vi "EnqueueSub.vi"(5 "is valid (T)":bool, 6 "is last element (F)":bool, 7 "nonFull":refnum<k4>, 8 "element in":T1, 9 "size":i32, 10 "lastID":u32, 11 "SubChannel in":refnum<class "SubChannelCPU.lvclass">) -> (0 "element out":T1, 1 "count":i32, 2 "wait":bool, 3 "SubChannel out":refnum<class "SubChannelCPU.lvclass">, 4 "id":u32)   [LabVIEW 2019, in "MessengerM.lvlib" / "SubChannelCPU.lvclass"]
uses:
  SubChannelCPU.lvclass
  <resource>/ChannelSupport/_ChannelSupport/PipeLogic2/PipeLogic2.lvclass
  Element.ctl
  MessengerM.lvlib
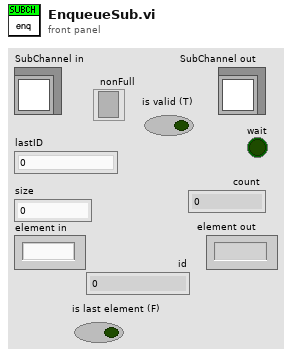
[diagram p1: front panel]
types:
  T1 = typedef "MessengerM.lvlib/Element.ctl" = string
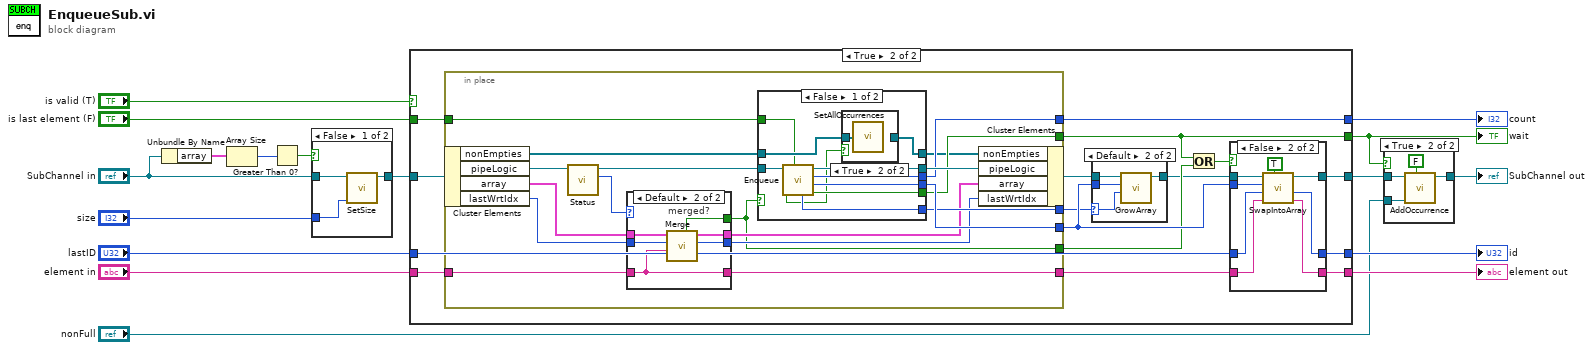
[diagram p0: block diagram]
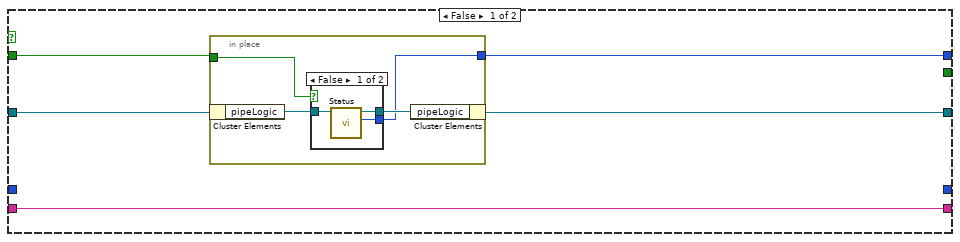
[diagram p2: hidden frame]
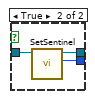
[diagram p3: hidden frame]
diagram:
  n1 = Unbundle By Name("SubChannel in") -> ("array"=w15:cluster{"elt":T1}[])
  n2 = Array Size(array=w15) -> (size(s)=w14:i32)
  n3 = Greater Than 0?(x=w14) -> (x > 0?=w16:bool)
  n4 = case shown="False" w16 {
    tunnel: "SubChannel in" -> [w20 w21]
    tunnel: [w19 w21] -> w17
    tunnel: "size" -> [w18 _]
    frame False {
      n5 = call "SetSize.vi"("size"=w18, "SubChannel in"=w20) -> ("SubChannel out"=w19:refnum<class "SubChannelCPU.lvclass">)  [unwired: 9 in]
    }
    frame True {
    }
  }
  n6 = case shown="True" "is valid (T)" {
    tunnel: w17 -> [w25 w51]
    tunnel: "element in" -> [w26 w44]
    tunnel: [w26 w43] -> w11
    tunnel: [w22 w42] -> w10
    tunnel: "lastID" -> [_ w41]
    tunnel: [_ w40] -> w8
    tunnel: [w24 w39] -> w7
    tunnel: [_ w38] -> w3
    tunnel: "is last element (F)" -> [w23 w37]
    frame False {
      n7 = in-place {
        in-place-border: w23 -> [w30]
        in-place-border: [w27] -> w22
        n8 = in-place-cluster #1(w25) -> ("pipeLogic"=w29:refnum<class "PipeLogic2.lvclass">)
        n9 = case shown="False" w30 {
          tunnel: w29 -> [w33 w36]
          tunnel: [w32 w35] -> w28
          tunnel: [w31 w34] -> w27
          frame False {
            n10 = call <resource>:"Status.vi"("pipeLogic in"=w33) -> ("count"=w31:i32, "pipeLogic out"=w32:refnum<class "PipeLogic2.lvclass">)  [unwired: 4 in, 5 out]
          }
          frame True {
            n11 = call <resource>:"SetSentinel.vi"("pipeLogic in"=w36) -> ("count"=w34:i32, "pipeLogic out"=w35:refnum<class "PipeLogic2.lvclass">)  [unwired: 8 in, 1 out]
          }
        }
        n12 = in-place-cluster #1("pipeLogic"=w28) -> (w24:refnum<class "SubChannelCPU.lvclass">)
      }
    }
    frame True {
      n13 = in-place {
        in-place-border: [w69] -> w42
        in-place-border: [w68] -> w52
        in-place-border: [w66] -> w47
        in-place-border: [w67] -> w38
        in-place-border: w44 -> [w60]
        in-place-border: [w59] -> w48
        in-place-border: [w56] -> w50
        in-place-border: w37 -> [w53]
        n14 = in-place-cluster #2(w51) -> ("nonEmpties"=w55:refnum<k4>[], "pipeLogic"=w65:refnum<class "PipeLogic2.lvclass">, "array"=w61:cluster{"elt":T1}[], "lastWrtIdx"=w58:i32)
        n15 = call <resource>:"Status.vi"("pipeLogic in"=w65) -> ("count"=w63:i32, "pipeLogic out"=w64:refnum<class "PipeLogic2.lvclass">)  [unwired: 4 in, 5 out]
        n16 = case shown="Default" w63 {
          tunnel: [w73 w76] -> w62
          tunnel: w61 -> [w73 w79]
          tunnel: w60 -> [w72 w78]
          tunnel: [_ w75] -> w56
          tunnel: [w72 w78] -> w59
          tunnel: w58 -> [w71 w77]
          tunnel: [w71 w74] -> w57
          frame 0 {
          }
          frame Default {
            # "merged?"
            n17 = call "Merge.vi"("element in"=w78, "lastWrtIdx in"=w77, "array in"=w79) -> ("lastWrtIdx out"=w74:i32, "array out"=w76:cluster{"elt":T1}[], "merged?"=w75:bool)  [unwired: 6 in]
          }
        }
        n18 = case shown="False" w56 {
          tunnel: [w89 w93] -> w70
          tunnel: [w88 _] -> w69
          tunnel: [w87 _] -> w68
          tunnel: [w86 _] -> w67
          tunnel: [w85 _] -> w66
          tunnel: w64 -> [w84 w93]
          tunnel: w55 -> [w82 w92]
          tunnel: [w81 w92] -> w54
          tunnel: w53 -> [w80 _]
          frame False {
            n19 = call <resource>:"Enqueue.vi"("last element in"=w80, "pipeLogic in"=w84) -> ("wait"=w86:bool, "index"=w87:i32, "count"=w88:i32, "pipeLogic out"=w89:refnum<class "PipeLogic2.lvclass">, "grow"=w85:i32, "set nonempty"=w83:bool)  [unwired: 2 in, 2 out]
            n20 = case shown="True" w83 {
              tunnel: w82 -> [w90 w91]
              tunnel: [w90 _] -> w81
              frame False {
              }
              frame True {
                n21 = call "SetAllOccurrences.vi"("occurrences"=w91) -> ()
              }
            }
          }
          frame True {
          }
        }
        n22 = in-place-cluster #2("nonEmpties"=w54, "pipeLogic"=w70, "array"=w62, "lastWrtIdx"=w57) -> (w45:refnum<class "SubChannelCPU.lvclass">)
      }
      n23 = case shown="Default" w47 {
        selector: w47 -> [_ w96]
        tunnel: w45 -> [w94 w98]
        tunnel: [w94 w97] -> w46
        tunnel: w52 -> [_ w95]
        frame 0 {
        }
        frame Default {
          n24 = call "GrowArray.vi"("grow"=w96, "index"=w95, "SubChannel in"=w98) -> ("SubChannel out"=w97:refnum<class "SubChannelCPU.lvclass">)  [unwired: 8 in]
        }
      }
      n25 = Or(x=w38, y=w50) -> (x .or. y?=w49:bool)
      n26 = case shown="False" w49 {
        tunnel: [w100 w108] -> w39
        tunnel: [w101 w106] -> w43
        tunnel: w48 -> [w101 w107]
        tunnel: w46 -> [w100 w109]
        tunnel: [w99 w104] -> w40
        tunnel: w52 -> [_ w103]
        tunnel: w41 -> [w99 w102]
        frame True {
          # "wait"
        }
        frame False {
          n27 = call "SwapIntoArray.vi"("enq"=TRUE, "element in"=w107, "last id"=w102, "index"=w103, "SubChannel in"=w109) -> ("element out"=w106:T1, "id"=w104:u32, "SubChannel out"=w108:refnum<class "SubChannelCPU.lvclass">)  [unwired: 4 in]
        }
      }
    }
  }
  "element out" <- w11
  "wait" <- w3
  "count" <- w10
  "id" <- w8
  n28 = case shown="True" w3 {
    tunnel: w7 -> [w110 w114]
    tunnel: [w110 w113] -> w6
    tunnel: "nonFull" -> [_ w111]
    frame False {
    }
    frame True {
      n29 = call "AddOccurrence.vi"("nonEmpty"=FALSE, "occ"=w111, "SubChannel in"=w114) -> ("SubChannel out"=w113:refnum<class "SubChannelCPU.lvclass">)  [unwired: 8 in]
    }
  }
  "SubChannel out" <- w6
